vi "Configure Window.vi"(8 "Prompt":string, 9 "Button Label":string, 11 "Open File in":refnum<class "Open File.lvclass">) -> (3 "Open File out":refnum<class "Open File.lvclass">)   [LabVIEW 2018, in "Open File Actor.lvlib" / "Open File.lvclass"]
uses:
  Open File.lvclass
  Open File.lvclass/Open File.ctl
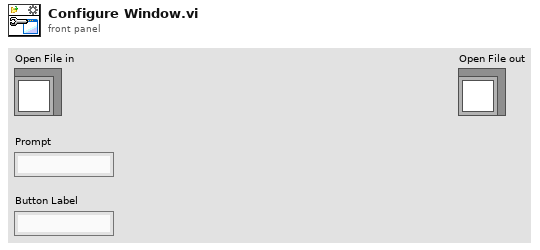
[diagram p1: front panel]
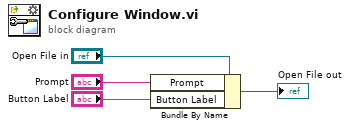
[diagram p0: block diagram]
diagram:
  n1 = Bundle By Name(cluster="Open File in", "Prompt"="Prompt", "Button Label"="Button Label") -> (→"Open File out":refnum<class "Open File.lvclass">)
